vi "Stop Process.vi"(8 "error in (no error)":errorcluster, 11 "DbgTimers in":refnum<class "DbgTimers.lvclass">) -> (0 "error out":errorcluster, 3 "DbgTimers out":refnum<class "DbgTimers.lvclass">)   [LabVIEW 2017, in "DbgTimers.lvclass"]
doc: "Developed by Kevin Thompson\nkevin@thompsonengineering.net\n\nCopyright 2018-2020\nThompson Engineering, LLC"
uses:
  DbgTimers.lvclass
  DbgTimers.lvclass/DbgTimers.ctl
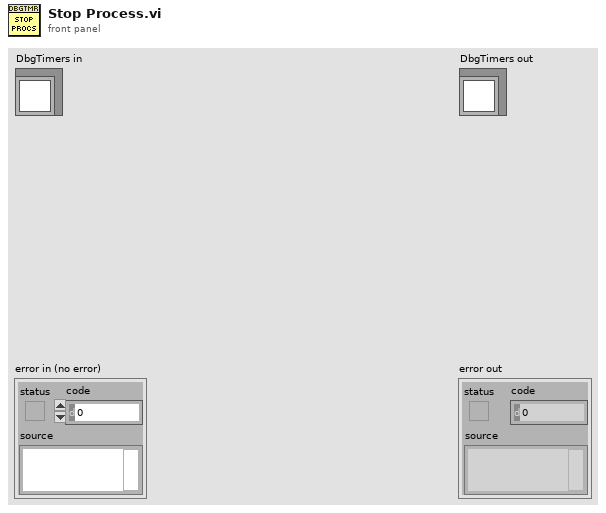
[diagram p1: front panel]
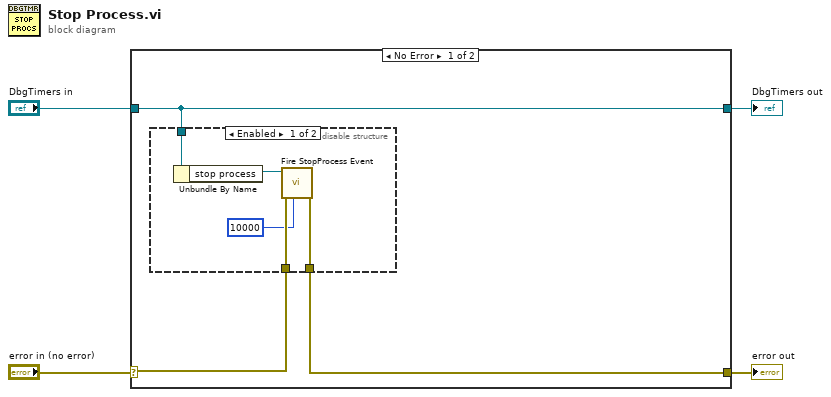
[diagram p0: block diagram]
diagram:
  n1 = case shown="No Error" "error in (no error)" {
    selector: "error in (no error)" -> [w6 w15]
    tunnel: [w5 w15] -> w3
    tunnel: [w7 w14] -> w1
    tunnel: "DbgTimers in" -> [w7 w14]
    frame No Error {
      n2 = disable-structure shown="Enabled" {
        disable-tunnel: w7 -> [w12 _]
        disable-tunnel: w6 -> [w9 w13]
        disable-tunnel: [w10 w13] -> w5
        frame Enabled {
          n3 = Unbundle By Name(w12) -> ("stop process"=w11:refnum<user-event>)
          n4 = call "Fire StopProcess Event.vi"("timeout in ms (5000)"=10000, "error in (no error)"=w9, "Event in"=w11) -> ("error out"=w10:errorcluster)  [unwired: 5 in, 3 out]
        }
        frame Disabled {
        }
      }
    }
    frame Error {
    }
  }
  "error out" <- w3
  "DbgTimers out" <- w1
